vi "Destroy Registry.vi"(8 "error in":errorcluster) -> (0 "error out":errorcluster)   [LabVIEW 2019, in "Identifier.lvclass"]
uses:
  Identifier.lvclass
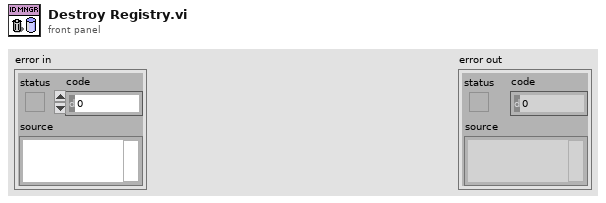
[diagram p1: front panel]
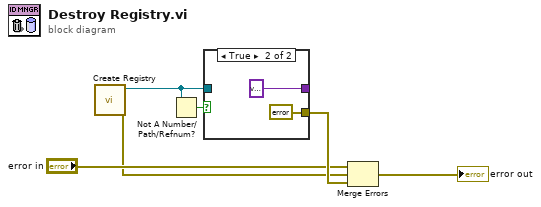
[diagram p0: block diagram]
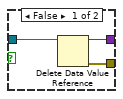
[diagram p2: hidden frame]
diagram:
  n1 = call "Create Registry.vi"() -> ("error out"=w1:errorcluster, "Registry"=w2:refnum<data-value>)  [unwired: 10 in]
  n2 = Not A Number/Path/Refnum?(number/path/refnum=w2) -> (NaN/Path/Refnum?=w6:bool)
  n3 = case shown="True" w6 {
    tunnel: w2 -> [w9 _]
    tunnel: [w7 errorcluster {"status"=FALSE, "code"=0, "source"=""} ("error out")] -> w5
    tunnel: [w8 variant] -> _
    frame False {
      n4 = Delete Data Value Reference(data value reference=w9) -> (data value=w8:variant, error out=w7:errorcluster)  [unwired: 1 in]
    }
    frame True {
    }
  }
  n5 = Merge Errors("error in", w1, w5) -> (→"error out":errorcluster)
